vi "1.1signal_sinus_flitré_level01.vi"() -> ()   [LabVIEW 2018]
uses:
  <vilib>/measure/maspectr.llb/FFT Spectrum (Mag-Phase) for 1 Chan.vi
  <vilib>/Analysis/3filter.llb/Butterworth Filter (DBL).vi
  <vilib>/measure/NI_MABase.lvlib
  <vilib>/Analysis/NI_AALBase.lvlib
  <vilib>/measure/NI_MAPro.lvlib
panel:
  out "signal x(t)":waveform(dbl)(graph)
  out "Spectre de x(t)":cluster{"f0":dbl, "df":dbl, "magnitude":dbl[]}(graph)
  out "Spectre de signal bruité":cluster{"f0":dbl, "df":dbl, "magnitude":dbl[]}(graph)
  out "signal x(t)+bruit":dbl[](graph)
  out "Spectre de Signal Aprés Filtrage":cluster{"f0":dbl, "df":dbl, "magnitude":dbl[]}(graph)
  out "Signal Aprés Filtrage":waveform(dbl)(graph)
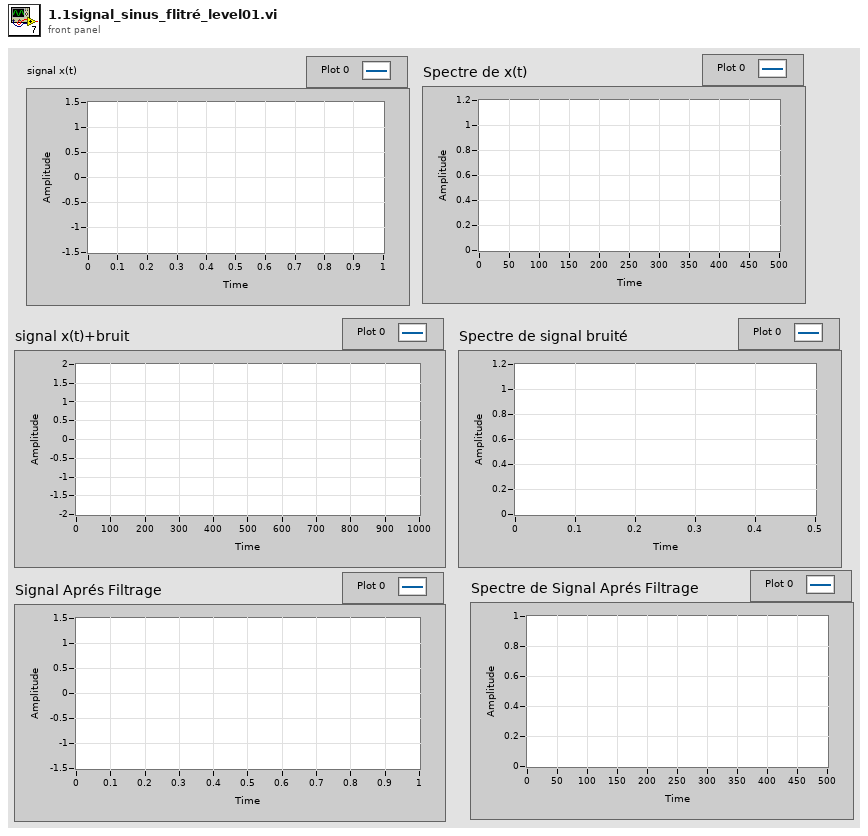
[diagram p1: front panel]
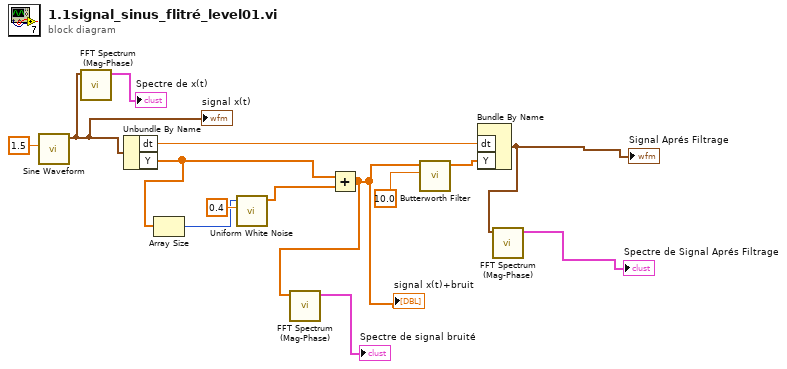
[diagram p0: block diagram]
diagram:
  n1 = call <vilib>:"Sine Waveform.vi"("amplitude"=1.5) -> ("signal out"=w1:waveform(dbl))  [unwired: 9 in, 1 out]
  "signal x(t)" <- w1
  n2 = call-poly <vilib>:"FFT Spectrum (Mag-Phase).vi"("time signal"=w1) -> ("magnitude"=→"Spectre de x(t)":cluster{"f0":dbl, "df":dbl, "magnitude":dbl[]})  [unwired: 6 in, 4 out]
  n3 = Unbundle By Name(w1) -> ("dt"=w9:dbl, "Y"=w10:dbl[])
  n4 = Array Size(array=w10) -> (size(s)=w12:i32)
  n5 = call <vilib>:"Uniform White Noise.vi"("amplitude"=0.4, "samples"=w12) -> ("uniform white noise"=w11:dbl[])  [unwired: 8 in, 1 out]
  n6 = Add(x=w10, y=w11) -> (x+y=w4:dbl[])
  "signal x(t)+bruit" <- w4
  n7 = call-poly <vilib>:"FFT Spectrum (Mag-Phase).vi"("time signal"=w4) -> ("magnitude"=→"Spectre de signal bruité":cluster{"f0":dbl, "df":dbl, "magnitude":dbl[]})  [unwired: 6 in, 4 out]
  n8 = call-poly <vilib>:"Butterworth Filter.vi"("sampling freq: fs"=10.0, "X"=w4) -> ("Filtered X"=w8:dbl[])  [unwired: 6 in, 1 out]
  n9 = Bundle By Name("dt"=w9, "Y"=w8) -> (w6:waveform(dbl))  [unwired: 1 in]
  "Signal Aprés Filtrage" <- w6
  n10 = call-poly <vilib>:"FFT Spectrum (Mag-Phase).vi"("time signal"=w6) -> ("magnitude"=→"Spectre de Signal Aprés Filtrage":cluster{"f0":dbl, "df":dbl, "magnitude":dbl[]})  [unwired: 6 in, 4 out]
